vi "Create Default Colors.vi"() -> (3 "Theme.Colors out":refnum<class "Theme.Colors.lvclass">)   [LabVIEW 2017, in "Theme.lvlib" / "Theme.Colors.lvclass"]
uses:
  Theme.Colors.lvclass
  Theme.Colors.lvclass/Theme.Colors.ctl
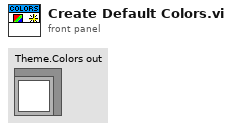
[diagram p1: front panel]
types:
  T1 = cluster{"Primary":u32, "Primary Variant":u32, "Secondary":u32, "Secondary Varient":u32}
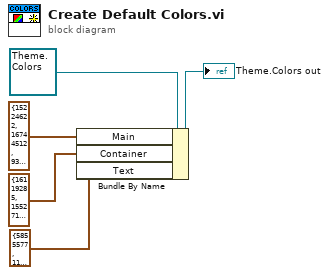
[diagram p0: block diagram]
diagram:
  n1 = Bundle By Name(cluster=refnum<class "Theme.Colors.lvclass"> refnum ("Theme.Colors in"), "Main"=T1 {"Primary"=15224622, "Primary Variant"=16744512, "Secondary"=9342606, "Secondary Varient"=2039583}, "Container"=cluster{"BG":u32, "Hover":u32, "Focused":u32} {"BG"=16119285, "Hover"=15527148, "Focused"=14474460}, "Text"=cluster{"Default":u32, "Error":u32} {"Default"=5855577, "Error"=11534368}) -> (→"Theme.Colors out":refnum<class "Theme.Colors.lvclass">)
